vi "RunNext.vi"(9 "Override":bool, 10 "Default":string, 11 "Cluster":T1) -> (1 "output cluster":T1, 3 "NextAction":string)   [LabVIEW 2023]
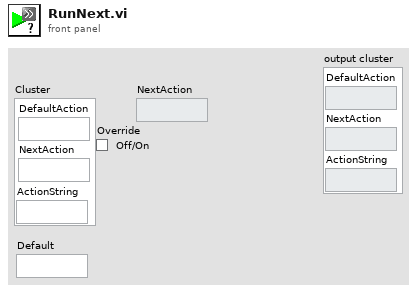
[diagram p1: front panel]
types:
  T1 = cluster{"DefaultAction":string, "NextAction":string, "ActionString":string}
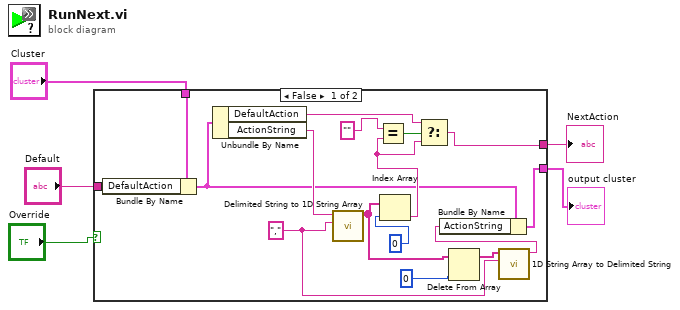
[diagram p0: block diagram]
diagram:
  n1 = case shown="False" "Override" {
    tunnel: [w21 w23] -> w5
    tunnel: "Default" -> [w20 w23]
    tunnel: "Cluster" -> [w19 w22]
    tunnel: [w11 w22] -> w2
    frame False {
      w8 = "," ("delimiter")
      n2 = Bundle By Name(cluster=w19, "DefaultAction"=w20) -> (w12:T1)
      n3 = Unbundle By Name(w12) -> ("DefaultAction"=w18:string, "ActionString"=w16:string)
      n4 = call <vilib>:"Delimited String to 1D String Array.vi"("delimiter"=w8, "delimited string"=w16) -> ("string array"=w10:string[])  [unwired: 9 in]
      n5 = Index Array(array=w10, index=0) -> (element=w13:string)
      n6 = Equal?(x="", y=w13) -> (x = y?=w17:bool)
      n7 = Select(t=w18, s=w17, f=w13) -> (s? t:f=w21:string)
      n8 = Delete From Array(array=w10, index=0) -> (array with subset deleted=w7:string[])  [unwired: 1 in, 1 out]
      n9 = call <vilib>:"1D String Array to Delimited String.vi"("delimiter"=w8, "string array"=w7) -> ("delimited string"=w6:string)  [unwired: 9 in]
      n10 = Bundle By Name(cluster=w12, "ActionString"=w6) -> (w11:T1)
    }
    frame True {
    }
  }
  "NextAction" <- w5
  "output cluster" <- w2
